vi "Get Encoder Info.vi"(8 "error in (no error)":errorcluster, 11 "CIPC Reference":u64) -> (0 "error out":errorcluster, 3 "Encoder Info":T1)   [LabVIEW 2021, in "CIF_NI_CIPC.lvlib"]
uses:
  CIF_NI_CIPC.lvlib
  TypeDefs/Encoder Info.ctl
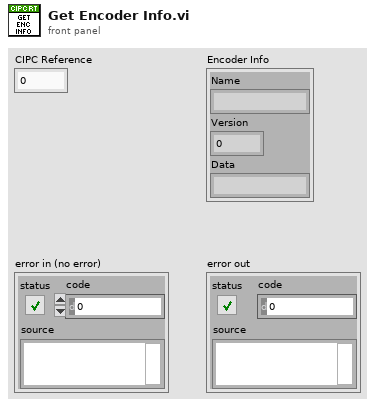
[diagram p1: front panel]
types:
  T1 = typedef "CIF_NI_CIPC.lvlib/Encoder Info.ctl" = cluster{"Name":string, "Version":i32, "Data":string}
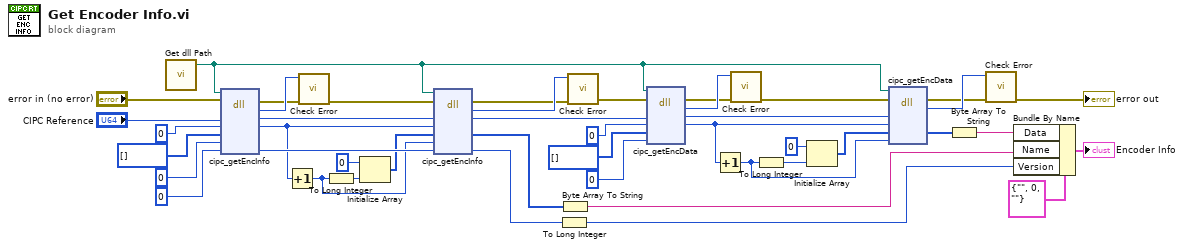
[diagram p0: block diagram]
diagram:
  n1 = call "Get dll Path.vi"() -> ("appended path"=w1:path)  [unwired: 5 in]
  n2 = dll-call lib="libnicipc.*" fn="cipc_getEncInfo"(path in=w1, error in="error in (no error)", "cipc_buffer_ref"="CIPC Reference", "enc_name_size"=u32 0 ("descr_size"), "enc_name"=u8[] [] ("initialized array"), "enc_name_maxsize"=u32 0 ("el_descr_maxsize"), "enc_version"=u32 0 ("head")) -> (error out=w43:errorcluster, "return type"=w44:i32, "cipc_buffer_ref"=w39:u64, "enc_name_size"=w35:u32, "enc_version"=w36:u32)  [unwired: 3 in, 1 out]
  n3 = Increment(x=w35) -> (x+1=w34:u32)
  n4 = call "Check Error.vi"("error in (no error)"=w43, "Error Code"=w44) -> ("error out"=w40:errorcluster)  [unwired: 9 in]
  n5 = To Long Integer(number=w34) -> (32bit integer=w8:i32)
  n6 = Initialize Array(u8 0, w8) -> (w32:u8[])
  n7 = dll-call lib="libnicipc.*" fn="cipc_getEncInfo"(path in=w1, error in=w40, "cipc_buffer_ref"=w39, "enc_name_size"=w35, "enc_name"=w32, "enc_name_maxsize"=w34, "enc_version"=w36) -> (error out=w41:errorcluster, "return type"=w42:i32, "cipc_buffer_ref"=w10:u64, "enc_name"=w31:u8[], "enc_version"=w33:u32)  [unwired: 3 in, 1 out]
  n8 = To Long Integer(number=w33) -> (32bit integer=w4:i32)
  n9 = Byte Array To String(unsigned byte array=w31) -> (string=w5:string)
  n10 = call "Check Error.vi"("error in (no error)"=w41, "Error Code"=w42) -> ("error out"=w9:errorcluster)  [unwired: 9 in]
  n11 = dll-call lib="libnicipc.*" fn="cipc_getEncData"(path in=w1, error in=w9, "cipc_buffer_ref"=w10, "enc_data_size"=u32 0 ("descr_size"), "enc_data"=u8[] [] ("initialized array"), "enc_data_maxsize"=u32 0 ("el_descr_maxsize")) -> (error out=w24:errorcluster, "return type"=w25:i32, "cipc_buffer_ref"=w20:u64, "enc_data_size"=w16:u32)  [unwired: 3 in, 1 out]
  n12 = Increment(x=w16) -> (x+1=w15:u32)
  n13 = call "Check Error.vi"("error in (no error)"=w24, "Error Code"=w25) -> ("error out"=w21:errorcluster)  [unwired: 9 in]
  n14 = To Long Integer(number=w15) -> (32bit integer=w7:i32)
  n15 = Initialize Array(u8 0, w7) -> (w14:u8[])
  n16 = dll-call lib="libnicipc.*" fn="cipc_getEncData"(path in=w1, error in=w21, "cipc_buffer_ref"=w20, "enc_data_size"=w16, "enc_data"=w14, "enc_data_maxsize"=w15) -> (error out=w22:errorcluster, "return type"=w23:i32, "enc_data"=w13:u8[])  [unwired: 4 in, 1 out]
  n17 = Byte Array To String(unsigned byte array=w13) -> (string=w11:string)
  n18 = call "Check Error.vi"("error in (no error)"=w22, "Error Code"=w23) -> ("error out"=→"error out":errorcluster)  [unwired: 9 in]
  n19 = Bundle By Name(cluster=T1 {"Name"="", "Version"=0, "Data"=""} ("Encoder Info 2"), "Data"=w11, "Name"=w5, "Version"=w4) -> (→"Encoder Info":T1)
